vi "TickTock (Testing).vi"(1 "EntryTick":u32, 2 "error in (no error)":errorcluster) -> (5 "Entry Diff":u32, 6 "Tick out":u32, 7 "error out":errorcluster, 8 "Last Call Diff":u32)   [LabVIEW 2014]
doc: "Use this VI as a FGV, or manual entry, tick counter to time VI execution. Wire the error clusters through this VI then read from the Diff outputs.\n\nLast Call Diff: Diff between last call tick value and current tick count.\nEntry Diff: Diff between Entry Tick value and current tick count."
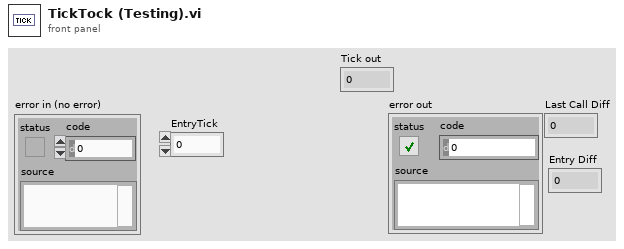
[diagram p1: front panel]
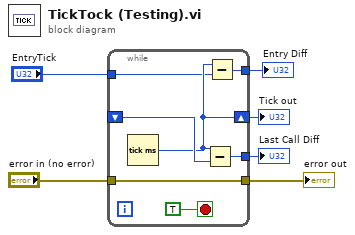
[diagram p0: block diagram]
diagram:
  n1 = while {
    tunnel: [w12] -> w6
    tunnel: "error in (no error)" -> [w12]
    shift-right: [w9] -> w1
    shift-left: _ -> [w11]
    tunnel: [w10] -> w5
    tunnel: "EntryTick" -> [w8]
    tunnel: [w7] -> w3
    stop <- TRUE stop-if-true
    n2 = Tick Count (ms)() -> (millisecond timer value=w9:u32)
    n3 = Subtract(x=w9, y=w11) -> (x-y=w10:u32)
    n4 = Subtract(x=w9, y=w8) -> (x-y=w7:u32)
  }
  "error out" <- w6
  "Last Call Diff" <- w5
  "Entry Diff" <- w3
  "Tick out" <- w1
